vi "GT_GetDo.vi"(10 "doType":u16(ring) items=["MC_ENABLE"=10, "MC_CLEAR"=11, "MC_GPO"=12], 11 "rtn_In":cluster{"rtn":i16, "Func":string}) -> (1 "IO":bool[](array[boolean]), 2 "doType":i16, 3 "rtn_Out":cluster{"rtn":i16, "Func":string})   [LabVIEW 2014]
uses:
  VC6/gts.dll
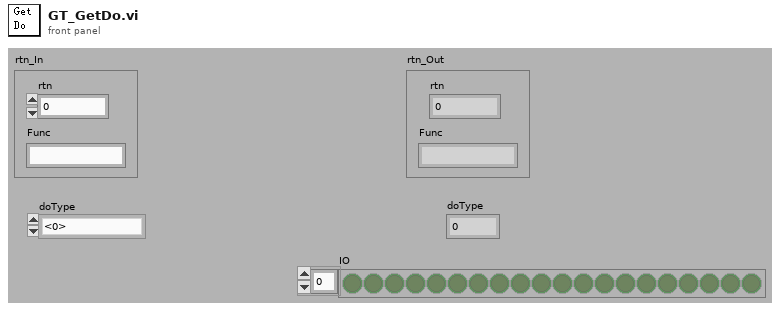
[diagram p1: front panel]
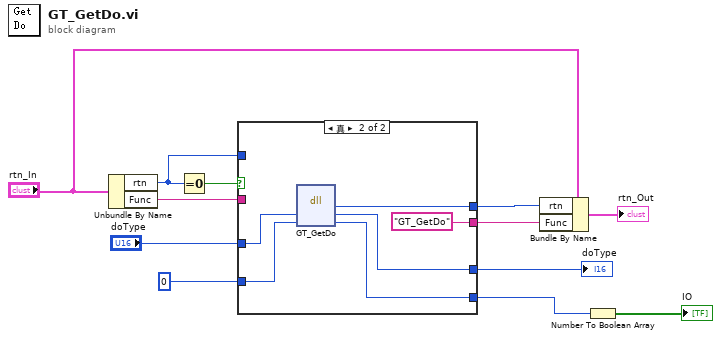
[diagram p0: block diagram]
diagram:
  n1 = Unbundle By Name("rtn_In") -> ("rtn"=w4:i16, "Func"=w3:string)
  n2 = Equal To 0?(x=w4) -> (x = 0?=w12:bool)
  n3 = case shown="真" w12 {
    tunnel: [w16 w22] -> w9
    tunnel: [w15 "GT_GetDo"] -> w8
    tunnel: "doType" -> [w14 w20]
    tunnel: 0 ("pValue") -> [w13 w19]
    tunnel: [w14 w18] -> w5
    tunnel: [w13 w17] -> w2
    tunnel: w4 -> [w16 _]
    tunnel: w3 -> [w15 _]
    frame False {
    }
    frame True {
      n4 = dll-call lib="PTH2Fabs DNewGTS AC-800LWin7版源程序-20170926gts85VC6gts.dll" fn="GT_GetDo"("doType"=w20, "pValue"=w19) -> ("rtn"=w22:i16, "doType"=w18:i16, "pValue"=w17:i32)  [unwired: 3 in, 2 out]
    }
  }
  "doType" <- w5
  n5 = Bundle By Name(cluster="rtn_In", "rtn"=w9, "Func"=w8) -> (→"rtn_Out":cluster{"rtn":i16, "Func":string})
  n6 = Number To Boolean Array(number=w2) -> (Boolean array=→"IO":bool[])
